vi "Test Generate Waveforms.vi"(8 "error in (no error)":errorcluster, 11 "Generator in":refnum<class "Generator.lvclass">) -> (0 "error out":errorcluster, 3 "Generator in":refnum<class "Generator.lvclass">)   [LabVIEW 2019, in "Generator.lvclass"]
uses:
  Generator.lvclass
  typedefs/AO.Channel--Cluster--Array.ctl
  typedefs/AO.Channel--Cluster.ctl
  typedefs/AO.Channel.Function--Enum.ctl
  typedefs/Sweep.Configuration--Cluster.ctl
  typedefs/Sweep.Channel--Cluster--Array.ctl
  typedefs/Sweep.Channel--Cluster.ctl
  typedefs/Sweep.Pattern--Enum.ctl
  typedefs/Sweep.State--enum.ctl
  Generator.lvclass/Generator.ctl
panel:
  out "Intensity Graph":dbl[][](graph)
  out "sweep state out":T1
  in  "Sweep Pattern":cluster{"Channel":u16, "Sweep Pattern":dbl[]}[](array[cluster])=[{"Channel"=1, "Sweep Pattern"=[0.0, 0.0, 0.01, 0.01, -0.01, -0.01, 0.0, 0.0]}] {"Sweep Pattern" format="%#_3p"; "Channel" min=1 max=128}
  in  "milliseconds to wait":u32=10
  out "Updates":i32=36
  out "Waveform Graph":waveform(dbl)[](graph)
  in  "Configuration.Sweep":T2={"Sweep Time (s)"=5.0, "Initial Wait (s)"=0.0, "Return to Start"=FALSE, "Channels"=[{"Enable?"=TRUE, "Channel"=1, "Start"=0.0, "End"=0.1, "Pattern"=enum."Table", "Table"=[]}]} {"Channels"."Table" format="%#_1f"; "Channels"."Channel" min=1 max=128; "Channels"."Start" format="%#_6p"; "Channels"."End" format="%#_6p"}
  in  "sampling":cluster{"Fs":dbl, "#s":i32}={"Fs"=55000.0, "#s"=8000} {"Fs" format="%#_13g"}
  in  "stop":bool
  in  "AO Channels":T6=[{"Enable?"=FALSE, "Channel"=0, "Amplitude"=0.001, "Offset"=0.0, "Frequency"=10.0, "Phase"=0.0, "Function"=enum."Sine", "Sweeping?"=FALSE, "Limit AC"=FALSE, "Limit DC?"=FALSE}] {"Phase" format="%.2g"; "Frequency" min=0.0001 max=10000.0 format="%.2g"; "Offset" format="%5.2p"; "Amplitude" min=0.0 max=10.0 format="%5.2p"}
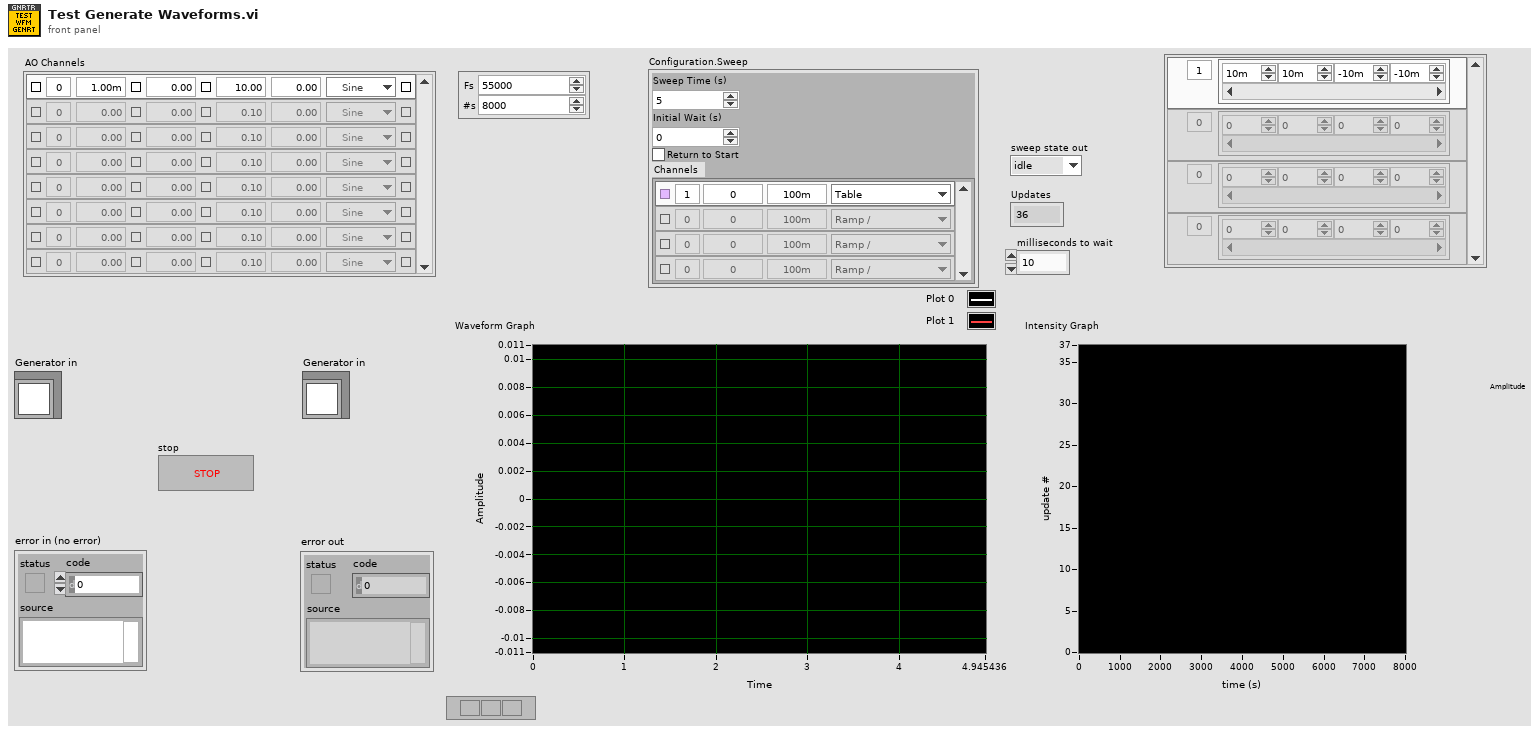
[diagram p1: front panel]
types:
  T1 = typedef "Generator.lvclass/Sweep.State--enum.ctl" = enum16{"idle", "initialize", "wait", "sweep", "stop"}
  T2 = typedef "Generator.lvclass/Sweep.Configuration--Cluster.ctl" = cluster{"Sweep Time (s)":dbl, "Initial Wait (s)":dbl, "Return to Start":bool, "Channels":T3}
  T3 = typedef "Generator.lvclass/Sweep.Channel--Cluster--Array.ctl" = T4[]
  T4 = typedef "Generator.lvclass/Sweep.Channel--Cluster.ctl" = cluster{"Enable?":bool, "Channel":u16, "Start":dbl, "End":dbl, "Pattern":T5, "Table":dbl[]}
  T5 = typedef "Generator.lvclass/Sweep.Pattern--Enum.ctl" = enum16{"Ramp /", "Ramp /\\", "Smooth Ramp _/", "Smooth Ramp _/\\_", "Table"}
  T6 = typedef "Generator.lvclass/AO.Channel--Cluster--Array.ctl" = T7[]
  T7 = typedef "Generator.lvclass/AO.Channel--Cluster.ctl" = cluster{"Enable?":bool, "Channel":i32, "Amplitude":dbl, "Offset":dbl, "Frequency":dbl, "Phase":dbl, "Function":T8, "Sweeping?":bool, "Limit AC":bool, "Limit DC?":bool}
  T8 = typedef "Generator.lvclass/AO.Channel.Function--Enum.ctl" = enum16{"Sine", "Triangle", "Square"}
  T9 = cluster{"AO":waveform(dbl)[], "REF_X":waveform(dbl)[], "REF_Y":waveform(dbl)[]}
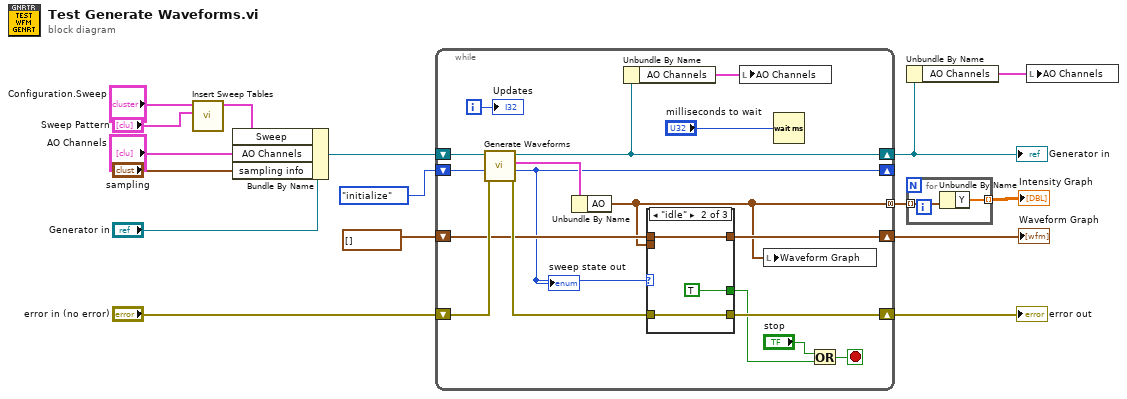
[diagram p0: block diagram]
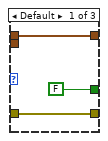
[diagram p2: hidden frame]
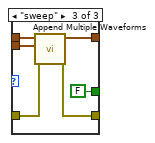
[diagram p3: hidden frame]
diagram:
  n1 = call "Insert Sweep Tables.vi"("Channels New"="Sweep Pattern", "Sweep Configuration in"="Configuration.Sweep") -> ("Sweep Configuration out"=w11:T2)  [unwired: 9 in]
  n2 = Bundle By Name(cluster="Generator in", "Sweep"=w11, "AO Channels"="AO Channels", "sampling info"="sampling") -> (w6:refnum<class "Generator.lvclass">)
  n3 = while {
    shift-right: [w32] -> w16
    shift-left: "error in (no error)" -> [w33]
    shift-right: [w25] -> w8
    shift-left: w6 -> [w31]
    shift-right: [w22] -> w3
    shift-left: waveform(dbl)[] [] ("Waveform out []") -> [w24]
    tunnel: [w19] -> w2 mode=concatenating
    shift-right: [w17] -> _
    shift-left: Sweep.State--enum."initialize" ("sweep state") -> [w18]
    i -> [w30]
    stop <- w29 stop-if-true
    n4 = call "Generate Waveforms.vi"("error in (no error)"=w33, "sweep state"=w18, "Generator.lvclass"=w31) -> ("error out"=w26:errorcluster, "sweep state out"=w17:T1, "Waveforms"=w23:T9, "Generator.lvclass"=w25:refnum<class "Generator.lvclass">)  [unwired: 5 in]
    "sweep state out" <- w17
    n5 = Unbundle By Name(w23) -> ("AO"=w19:waveform(dbl)[])
    n6 = Unbundle By Name(w25) -> ("AO Channels"=w27:T6)
    n7 = case shown="\"idle\"" w17 {
      tunnel: [w35 w38 w45] -> w32
      tunnel: w26 -> [w35 w38 w44]
      tunnel: w19 -> [_ _ w43]
      tunnel: w24 -> [w36 w39 w42]
      tunnel: [w36 w39 w41] -> w22
      tunnel: [FALSE TRUE FALSE] -> w20
      frame Default {
      }
      frame "idle" {
      }
      frame "sweep" {
        n8 = call "Append Multiple Waveforms.vi"("error in (no error)"=w44, "Waveform B []"=w43, "Waveforrm A []"=w42) -> ("error out"=w45:errorcluster, "Waveform out []"=w41:waveform(dbl)[])  [unwired: 7 in]
      }
    }
    n9 = local write "AO Channels"(w27) -> ()
    n10 = local write "Waveform Graph"(w19) -> ()
    n11 = Wait (ms)(milliseconds to wait="milliseconds to wait") -> ()  [unwired: 1 out]
    n12 = Or(x="stop", y=w20) -> (x .or. y?=w29:bool)
    "Updates" <- w30
  }
  "error out" <- w16
  "Generator in" <- w8
  "Waveform Graph" <- w3
  n13 = Unbundle By Name(w8) -> ("AO Channels"=w9:T6)
  n14 = for {
    tunnel: w2 -> [w47] mode=indexing
    tunnel: [w46] -> w1 mode=indexing
    n15 = Unbundle By Name(w47) -> ("Y"=w46:dbl[])
  }
  "Intensity Graph" <- w1
  n16 = local write "AO Channels"(w9) -> ()
